vi "Convert_to_2009.vi"(8 "error in (no error)":errorcluster, 10 "2009 data in":T1={"DistSettings"={"BuildLabel"="", "ProductName"="", "BuildLocation"=path "", "MediaSize"=0, "Language"=9, "ProductVersion"={"Major"=1, "Minor"=0, "Update"=0}, "AutoIncrement"=FALSE, "ReadmeID"="", "LicenseID"="", "arpCompany"="", "arpURL"="http://", "arpContact"="", "arpPhone"="", "Executable"="", "CmdArg"="", "OSCheck"=0, "Hide"=FALSE, "LV80higher"=FALSE, "IncludeError?"=FALSE, "HWOption"=enum."<none>", "HWPath"=path "", "UpgradeCode"="", "Author"="", "MsiFileName"="", "CabFileName"="", "DistID"="", "WindowTitle"="", "WindowMessage"="", "CacheDistros"=FALSE, "EXE str ref?"=FALSE}, "BldInfo"=[], "FileInfo"=[], "DirInfo"=[], "ShortcutInfo"=[], "RegInfo"=[], "RegData"=[], "DistParts"=[], "DefaultDir"=""} {"RegData"."Values"."Type" items=["Bare", "String", "Expandable String", "Binary", "DWord"]; "DistSettings"."ProductVersion"."Update" step=1; "DistSettings"."ProductVersion"."Minor" step=1; "DistSettings"."ProductVersion"."Major" step=1; "DistSettings"."Language" items=["English"=9, "German"=7, "French"=12, "Japanese"=17, "Korean"=18, "Chinese (Simplified)"=2052]}, 11 "IB_Source in":refnum<class "IB_Source.lvclass">) -> (0 "error out":errorcluster, 2 "2009 data out":T1={"DistSettings"={"BuildLabel"="", "ProductName"="", "BuildLocation"=path "", "MediaSize"=0, "Language"=9, "ProductVersion"={"Major"=1, "Minor"=0, "Update"=0}, "AutoIncrement"=FALSE, "ReadmeID"="", "LicenseID"="", "arpCompany"="", "arpURL"="http://", "arpContact"="", "arpPhone"="", "Executable"="", "CmdArg"="", "OSCheck"=0, "Hide"=FALSE, "LV80higher"=FALSE, "IncludeError?"=FALSE, "HWOption"=enum."<none>", "HWPath"=path "", "UpgradeCode"="", "Author"="", "MsiFileName"="", "CabFileName"="", "DistID"="", "WindowTitle"="", "WindowMessage"="", "CacheDistros"=FALSE, "EXE str ref?"=FALSE}, "BldInfo"=[], "FileInfo"=[], "DirInfo"=[], "ShortcutInfo"=[], "RegInfo"=[], "RegData"=[], "DistParts"=[], "DefaultDir"=""} {"RegData"."Values"."Type" items=["Bare", "String", "Expandable String", "Binary", "DWord"]; "DistSettings"."ProductVersion"."Update" step=1; "DistSettings"."ProductVersion"."Minor" step=1; "DistSettings"."ProductVersion"."Major" step=1; "DistSettings"."Language" items=["English"=9, "German"=7, "French"=12, "Japanese"=17, "Korean"=18, "Chinese (Simplified)"=2052]})   [LabVIEW 2020, in "IB_Source.lvclass"]
uses:
  <vilib>/AppBuilder/IB_Classes/Source/IB_Source.lvclass
  <vilib>/AppBuilder/IB_Classes/Source/IB_Source.lvclass/IB_Source.ctl
  <resource>/Framework/Providers/Builds/Installer/CDK_sTypeDef_BuildInfo.ctl
  <resource>/Framework/Providers/Builds/Installer/CDK_sTypeDef_BuildTypes.ctl
  <resource>/Framework/Providers/Builds/Installer/CDK_sTypeDef_FileInfo.ctl
  <resource>/Framework/Providers/Builds/Installer/CDK_sTypeDef_ShortcutInfo.ctl
  <resource>/Framework/Providers/Builds/Installer/CDK_sTypeDef_DirInfo.ctl
  <resource>/Framework/Providers/Builds/Installer/CDK_sTypeDef_Languages.ctl
  <resource>/Framework/Providers/Builds/Installer/CDK_sTypeDef_ProductVersion.ctl
  <resource>/Framework/Providers/Builds/Installer/CDK_sTypeDef_HWImportOption.ctl
  <resource>/Framework/Providers/Builds/Installer/CDK_sTypeDef_DISTSETTINGS.ctl
  AppLibs/distkit/MDF/NIMdf.llb/MDFBDPRegKeyType.ctl
  AppLibs/distkit/MDF/NI_MDF.lvlib
  <resource>/Framework/Providers/Builds/Installer/CDK_sTypeDef_RegData.ctl
  <resource>/Framework/Providers/Builds/Installer/CDK_sTypeDef_DistParts.ctl
  <vilib>/AppBuilder/IB_RW_Project/Compatibility/CDK_sTypeDef_2009_data.ctl
  <resource>/Framework/Providers/Builds/Installer/CDK_sTypeDef_SoftDep.ctl
panel:
  # "."
  # "."
  # "."
  # "."
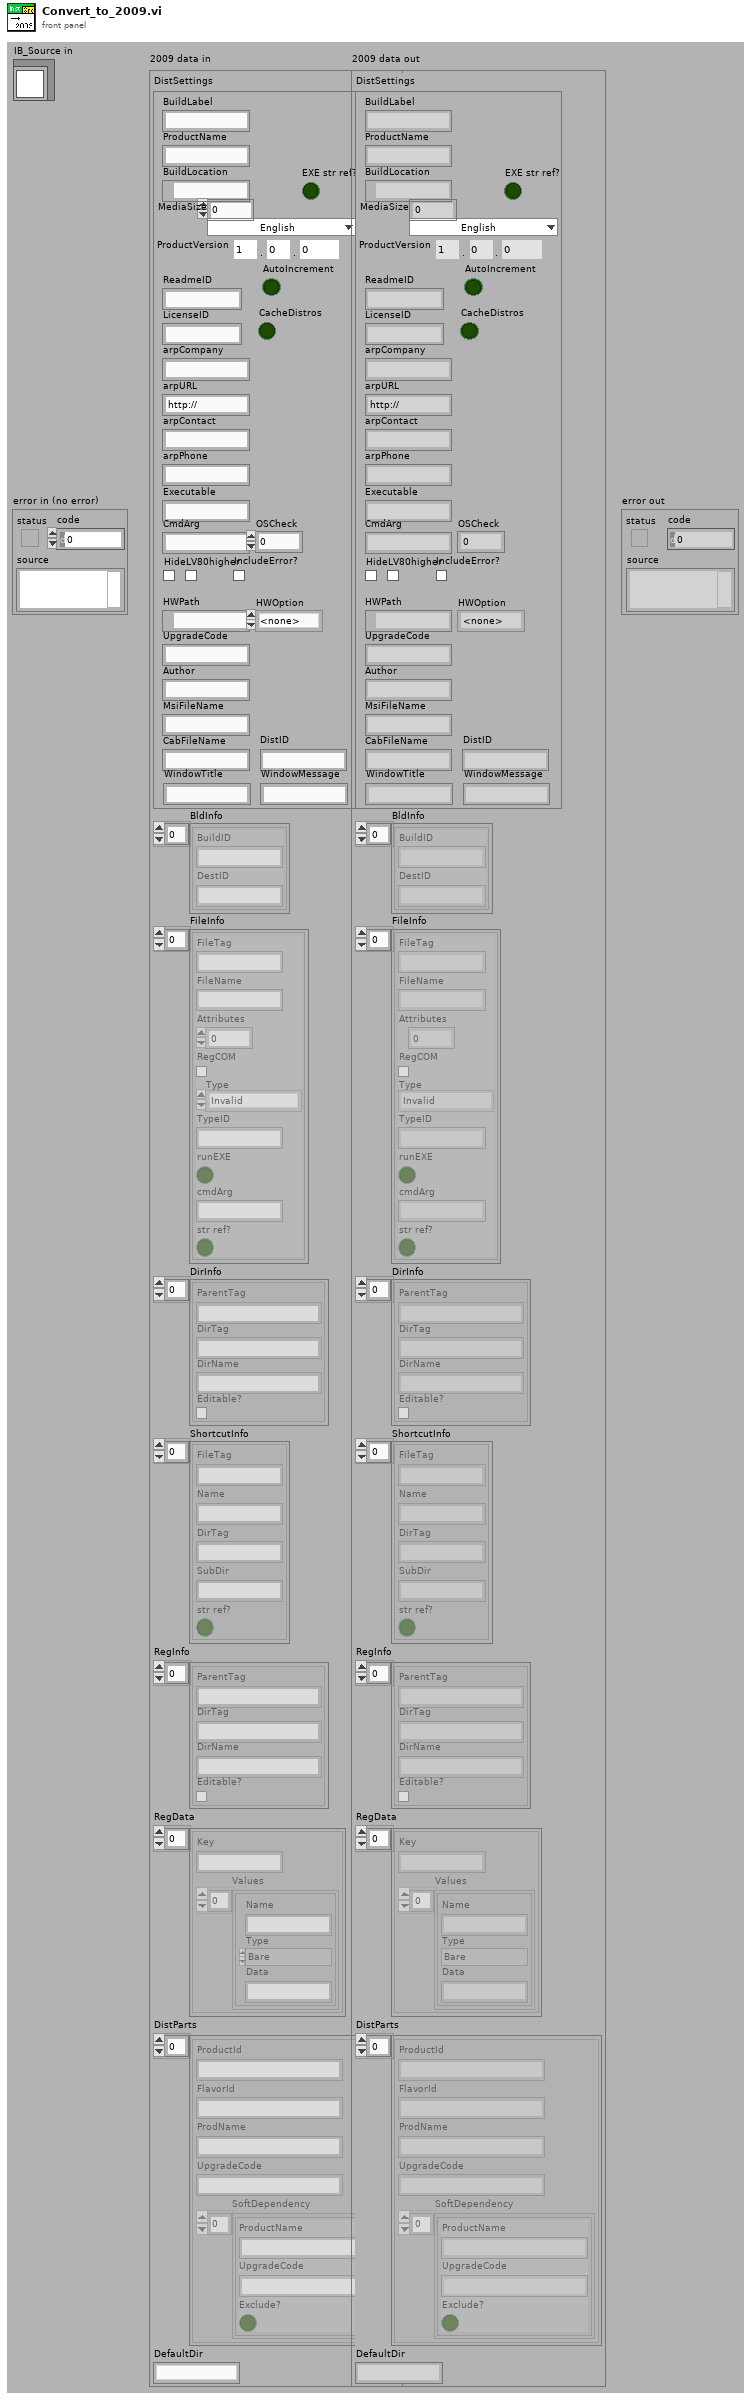
[diagram p1: front panel]
types:
  T1 = typedef "CDK_sTypeDef_2009_data.ctl" = cluster{"DistSettings":T2, "BldInfo":T6[], "FileInfo":T7[], "DirInfo":T9[], "ShortcutInfo":T10[], "RegInfo":T9[], "RegData":T11[], "DistParts":T13[], "DefaultDir":string}
  T2 = typedef "CDK_sTypeDef_DISTSETTINGS.ctl" = cluster{"BuildLabel":string, "ProductName":string, "BuildLocation":path, "MediaSize":u16, "Language":T3, "ProductVersion":T4, "AutoIncrement":bool, "ReadmeID":string, "LicenseID":string, "arpCompany":string, "arpURL":string, "arpContact":string, "arpPhone":string, "Executable":string, "CmdArg":string, "OSCheck":i32, "Hide":bool, "LV80higher":bool, "IncludeError?":bool, "HWOption":T5, "HWPath":path, "UpgradeCode":string, "Author":string, "MsiFileName":string, "CabFileName":string, "DistID":string, "WindowTitle":string, "WindowMessage":string, "CacheDistros":bool, "EXE str ref?":bool}
  T3 = typedef "CDK_sTypeDef_Languages.ctl" = u16
  T4 = typedef "CDK_sTypeDef_ProductVersion.ctl" = cluster{"Major":u8, "Minor":u8, "Update":u16}
  T5 = typedef "CDK_sTypeDef_HWImportOption.ctl" = enum16{"<none>", "Merge", "Replace", "Dialog"}
  T6 = typedef "CDK_sTypeDef_BuildInfo.ctl" = cluster{"BuildID":string, "DestID":string}
  T7 = typedef "CDK_sTypeDef_FileInfo.ctl" = cluster{"FileTag":string, "FileName":string, "Attributes":i16, "RegCOM":bool, "Type":T8, "TypeID":string, "runEXE":bool, "cmdArg":string, "str ref?":bool}
  T8 = typedef "CDK_sTypeDef_BuildTypes.ctl" = enum16{"Invalid", "File", "Folder", "BuildRule", "Library"}
  T9 = typedef "CDK_sTypeDef_DirInfo.ctl" = cluster{"ParentTag":string, "DirTag":string, "DirName":string, "Editable?":bool}
  T10 = typedef "CDK_sTypeDef_ShortcutInfo.ctl" = cluster{"FileTag":string, "Name":string, "DirTag":string, "SubDir":string, "str ref?":bool}
  T11 = typedef "CDK_sTypeDef_RegData.ctl" = cluster{"Key":string, "Values":cluster{"Name":string, "Type":T12, "Data":string}[]}
  T12 = typedef "NI_MDF.lvlib/MDFBDPRegKeyType.ctl" = i32
  T13 = typedef "CDK_sTypeDef_DistParts.ctl" = cluster{"ProductId":string, "FlavorId":string, "ProdName":string, "UpgradeCode":string, "SoftDependency":T14[]}
  T14 = typedef "CDK_sTypeDef_SoftDep.ctl" = cluster{"ProductName":string, "UpgradeCode":string, "Exclude?":bool}
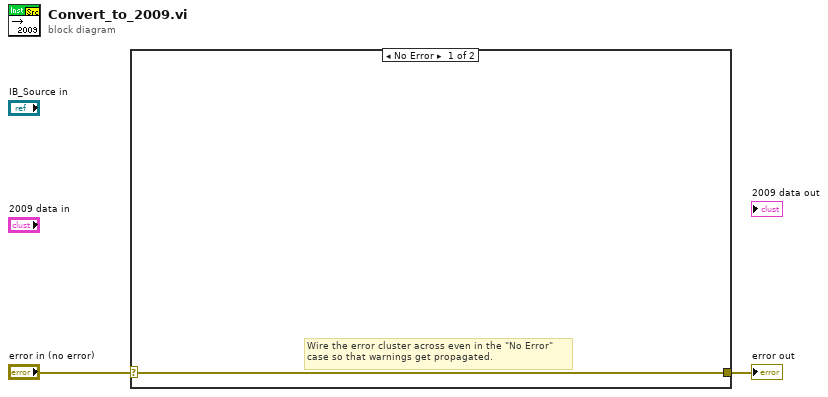
[diagram p0: block diagram]
diagram:
  n1 = case shown="No Error" "error in (no error)" {
    selector: "error in (no error)" -> [w3 w4]
    tunnel: [w3 w4] -> w1
    frame No Error {
      # "Wire the error cluster across even in the \"No Error\"\ncase so that warnings get propagated."
    }
    frame Error {
    }
  }
  "error out" <- w1
